vi "Get Module Type.vi"(8 "error in (no error)":errorcluster, 11 "IVI Refnum in":refnum<k15>) -> (0 "error out":errorcluster, 1 "timekeeper check error out":errorcluster, 2 "Module type":T1, 3 "IVI Refnum out":refnum<k15>)   [LabVIEW 2026, in "NI Synchronization Engine.lvlib"]
uses:
  NI Synchronization Engine.lvlib
  timekeeper type.ctl
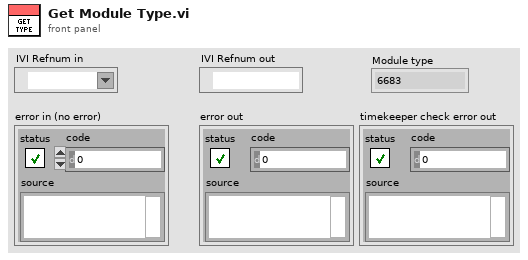
[diagram p1: front panel]
types:
  T1 = typedef "NI Synchronization Engine.lvlib/timekeeper type.ctl" = enum16{"6683", "6683H", "6682", "6682H", "non-timekeeper", "timekeeper"}
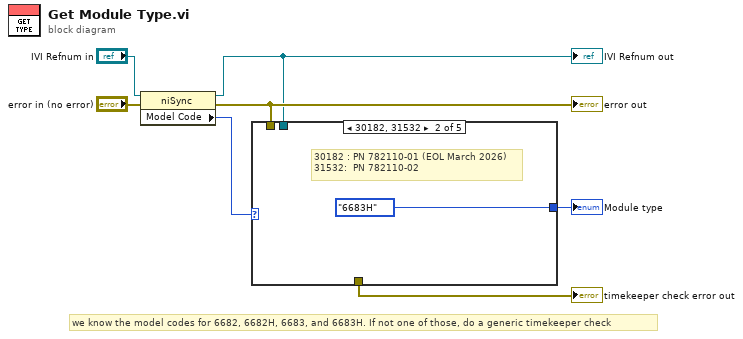
[diagram p0: block diagram]
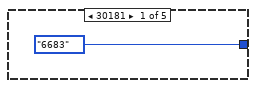
[diagram p2: hidden frame]
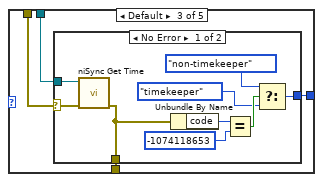
[diagram p3: hidden frame]
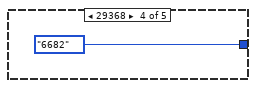
[diagram p5: hidden frame]
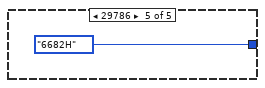
[diagram p6: hidden frame]
diagram:
  # "we know the model codes for 6682, 6682H, 6683, and 6683H. If not one of those, do a generic timekeeper check"
  n1 = property class="niSync"(reference="IVI Refnum in", error in="error in (no error)") -> (reference out=w3:refnum<k15>, error out=w4:errorcluster, "Model Code"=w5:i32)
  "IVI Refnum out" <- w3
  "error out" <- w4
  n2 = case shown="30182, 31532" w5 {
    tunnel: [timekeeper_type."6683" ("Timekeeper type") timekeeper_type."6683H" ("Timekeeper type") w10 timekeeper_type."6682" ("Timekeeper type") timekeeper_type."6682H" ("Timekeeper type")] -> w1
    tunnel: w4 -> [_ _ w13 _ _]
    tunnel: w3 -> [_ _ w12 _ _]
    tunnel: [_ _ w11 _ _] -> w2
    frame 30181 {
    }
    frame 30182, 31532 {
      # "30182 : PN 782110-01 (EOL March 2026)\n31532:  PN 782110-02"
    }
    frame Default {
      n3 = case shown="No Error" w13 {
        selector: w13 -> [w21 _]
        tunnel: w12 -> [w22 _]
        tunnel: [w16 _] -> w10
        tunnel: [w15 _] -> w11
        frame No Error {
          n4 = call <instrlib>:"niSync Get Time.vi"("error in (no error)"=w21, "instrument handle"=w22) -> ("error out"=w15:errorcluster)  [unwired: 5 in, 2 out]
          n5 = Unbundle By Name(w15) -> ("code"=w20:i32)
          n6 = Equal?(x=w20, y=-1074118653) -> (x = y?=w18:bool)
          n7 = Select(t=timekeeper_type."non-timekeeper" ("Timekeeper type"), s=w18, f=timekeeper_type."timekeeper" ("Timekeeper type")) -> (s? t:f=w16:T1)
        }
        frame Error {
        }
      }
    }
    frame 29368 {
    }
    frame 29786 {
    }
  }
  "Module type" <- w1
  "timekeeper check error out" <- w2
